vi "Read XNET.vi"(8 "error in":errorcluster, 11 "PCAN in":refnum<class "PCAN.lvclass">) -> (0 "error out":errorcluster, 3 "PCAN out":refnum<class "PCAN.lvclass">)   [LabVIEW 2024, in "PCAN.lvlib" / "PCAN.lvclass"]
uses:
  PCAN.lvclass
  PCAN.lvclass/PCAN.ctl
  <vilib>/xnet/xnet.llb/XNET Frame Type CAN.ctl
  <vilib>/xnet/xnet.llb/XNET Convert (Frame CAN to Signal).vi
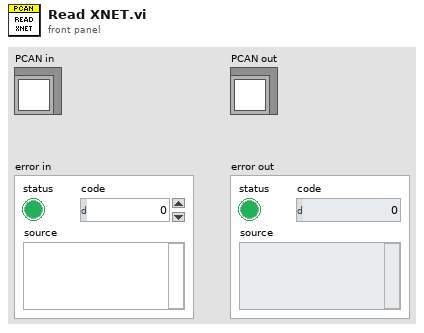
[diagram p1: front panel]
types:
  T1 = typedef "TPCANHandle.ctl" = enum16{"PCAN_NONEBUS  0x000", "PCAN_ISABUS1  0x21", "PCAN_ISABUS2  0x22", "PCAN_ISABUS3  0x23", "PCAN_ISABUS4  0x24", "PCAN_ISABUS5  0x25", "PCAN_ISABUS6  0x26", "PCAN_ISABUS7  0x27", "PCAN_ISABUS8  0x28", "PCAN_DNGBUS1  0x31", "PCAN_PCIBUS1  0x41", "PCAN_PCIBUS1  0x42", "PCAN_PCIBUS1  0x43", "PCAN_PCIBUS1  0x44", "PCAN_PCIBUS1  0x45", "PCAN_PCIBUS1  0x46", "PCAN_PCIBUS1  0x47", "PCAN_PCIBUS1  0x48", "PCAN_PCIBUS1  0x409", "PCAN_PCIBUS1  0x40A", "PCAN_PCIBUS1  0x40B", "PCAN_PCIBUS1  0x40C", "PCAN_PCIBUS1  0x40D", "PCAN_PCIBUS1  0x40E", "PCAN_PCIBUS1  0x40F", "PCAN_PCIBUS1  0x410", "PCAN_USBBUS1  0x51", "PCAN_USBBUS2  0x52", "PCAN_USBBUS3  0x53", "PCAN_USBBUS4  0x54", "PCAN_USBBUS5  0x55", "PCAN_USBBUS6  0x56", "PCAN_USBBUS7  0x57", "PCAN_USBBUS8  0x58", "PCAN_USBBUS9  0x509", "PCAN_USBBUS10  0x50A", "PCAN_USBBUS11  0x50B", "PCAN_USBBUS12  0x50C", "PCAN_USBBUS13  0x50D", "PCAN_USBBUS14  0x50E", "PCAN_USBBUS15  0x50F", "PCAN_USBBUS16  0x510", "PCAN_PCCBUS1  0x61", "PCAN_PCCBUS2  0x62", "PCAN_LANBUS1  0x801", "PCAN_LANBUS2  0x802", "PCAN_LANBUS3  0x803", "PCAN_LANBUS4  0x804", "PCAN_LANBUS5  0x805", "PCAN_LANBUS6  0x806", "PCAN_LANBUS7  0x807", "PCAN_LANBUS8  0x808", "PCAN_LANBUS9  0x809", "PCAN_LANBUS10  0x80A", "PCAN_LANBUS11  0x80B", "PCAN_LANBUS12  0x80C", "PCAN_LANBUS13  0x80D", "PCAN_LANBUS14  0x80E", "PCAN_LANBUS15  0x80F", "PCAN_LANBUS16  0x810"}
  T2 = typedef "TPCANTimestamp.ctl" = cluster{"millis overflow":u16, "millis ":u32, "micros":u16}
  T3 = typedef "CAN MSG Cluster.ctl" = cluster{"ID":u32, "MSG type":u8, "DLC":u8, "DATA":u8[]}
  T4 = typedef "XNET Frame Type CAN.ctl" = u8
  T5 = cluster{"timestamp":timestamp, "payload":u8[], "identifier":u32, "type":T4, "extended?":bool, "echo?":bool}
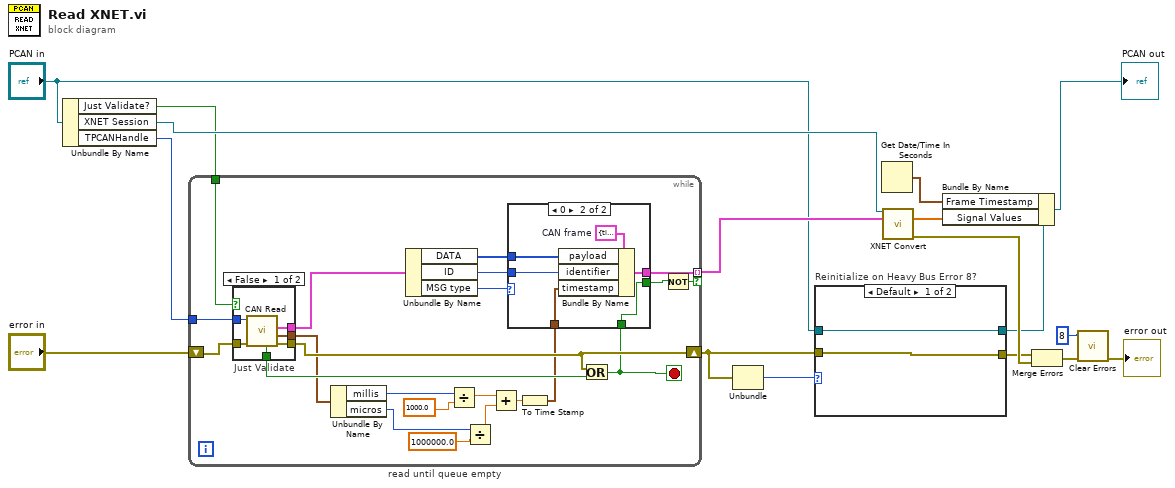
[diagram p0: block diagram]
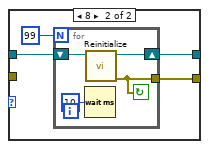
[diagram p2: hidden frame]
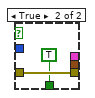
[diagram p3: hidden frame]
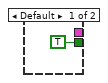
[diagram p4: hidden frame]
diagram:
  n1 = Unbundle By Name("PCAN in") -> ("Just Validate?"=w1:bool, "XNET Session"=w15:refnum<k21>, "TPCANHandle"=w14:T1)
  n2 = while "read until queue empty" {
    tunnel: w14 -> [w39]
    shift-right: [w36] -> w12
    shift-left: "error in" -> [w38]
    tunnel: [w22] -> w16 mode=indexing if=w35
    tunnel: w1 -> [w18]
    stop <- w19 stop-if-true
    n3 = case "Just Validate" shown="False" w18 {
      tunnel: w39 -> [w45 _]
      tunnel: w38 -> [w44 w47]
      tunnel: [w43 TRUE ("rcv queue empty")] -> w37
      tunnel: [w42 w47] -> w36
      tunnel: [w41 _] -> w34
      tunnel: [w40 _] -> w31
      frame False {
        n4 = call <instrlib>:"CAN Read.vi"("error in (no error)"=w44, "TPCANHandle"=w45) -> ("error out"=w42:errorcluster, "TPCANTimestamp out"=w40:T2, "CAN_Message out"=w41:T3, "rcv queue empty"=w43:bool)  [unwired: 5 in, 1 out]
      }
      frame True {
      }
    }
    n5 = Unbundle By Name(w31) -> ("millis"=w30:u32, "micros"=w28:u16)
    n6 = Unbundle By Name(w34) -> ("DATA"=w33:u8[], "ID"=w32:u32, "MSG type"=w21:u8)
    n7 = Divide(x=w30, y=1000.0) -> (x/y=w24:dbl)
    n8 = Divide(x=w28, y=1000000.0) -> (x/y=w25:dbl)
    n9 = Add(x=w24, y=w25) -> (x+y=w26:dbl)
    n10 = To Time Stamp(1:w26) -> (0:w23:timestamp)
    n11 = Or(x=w36, y=w37) -> (x .or. y?=w19:bool)
    n12 = case shown="0" w21 {
      tunnel: w33 -> [_ w53]
      tunnel: w32 -> [_ w52]
      tunnel: w23 -> [_ w51]
      tunnel: [_ w50] -> w22
      tunnel: [TRUE w49] -> w20
      tunnel: w19 -> [_ w49]
      frame Default {
      }
      frame 0 {
        w54 = T5 {"timestamp"=timestamp(0 s since 1904-01-01), "payload"=[], "identifier"=0, "type"=0, "extended?"=FALSE, "echo?"=FALSE}  # CAN frame
        n13 = Bundle By Name(cluster=w54, "payload"=w53, "identifier"=w52, "timestamp"=w51) -> (w50:T5)
      }
    }
    n14 = Not(x=w20) -> (.not. x?=w35:bool)
  }
  n15 = Unbundle(w12) -> ("code"=w13:i32)  [unwired: 2 out]
  n16 = case "Reinitialize on Heavy Bus Error 8?" shown="Default" w13 {
    tunnel: [w56 w60] -> w10
    tunnel: w12 -> [w56 _]
    tunnel: "PCAN in" -> [w55 w59]
    tunnel: [w55 w58] -> w7
    frame Default {
    }
    frame 8 {
      n17 = for {
        N: 99 -> [_]
        tunnel: [w62] -> w60
        shift-right: [w63] -> w58
        shift-left: w59 -> [w64]
        stop <- w62 continue-if-true
        n18 = Wait (ms)(milliseconds to wait=u32 10) -> ()  [unwired: 1 out]
        n19 = call "Reinitialize.vi"("PCAN in"=w64) -> ("error out"=w62:errorcluster, "PCAN out"=w63:refnum<class "PCAN.lvclass">)  [unwired: 9 in]
      }
    }
  }
  n20 = Get Date/Time In Seconds() -> (seconds since 1Jan1904=w3:timestamp)
  n21 = call-poly <vilib>:"XNET Convert.vi"("session in"=w15, "frame data"=w16) -> ("signal data"=w8:dbl[], "error out"=w11:errorcluster)  [unwired: 11 in, 1 out]
  n22 = Bundle By Name(cluster=w7, "Frame Timestamp"=w3, "Signal Values"=w8) -> (→"PCAN out":refnum<class "PCAN.lvclass">)
  n23 = Merge Errors(w10, w11) -> (w9:errorcluster)
  n24 = call <vilib>:"Clear Errors.vi"("error in (no error)"=w9, "specific error code to clear (0: all)"=8) -> ("error out"=→"error out":errorcluster)  [unwired: 4 in, 1 out]
